vi "(Sub) Falling Step.vi"(7 "State":T1(ring), 8 "error in (no error)":errorcluster caption="에러 입력(에러 없음)", 9 "G3. Rising Step":dbl[](array[numeric]), 10 "G2. Rising Step":dbl[](array[numeric]), 11 "G1. Rising Step":dbl[](array[numeric])) -> (0 "error out":errorcluster caption="에러 출력", 1 "G3. Falling Step":dbl[](array[numeric]), 2 "G2. Falling Step":dbl[](array[numeric]), 3 "G1. Falling Step":dbl[](array[numeric]))   [LabVIEW 2017]
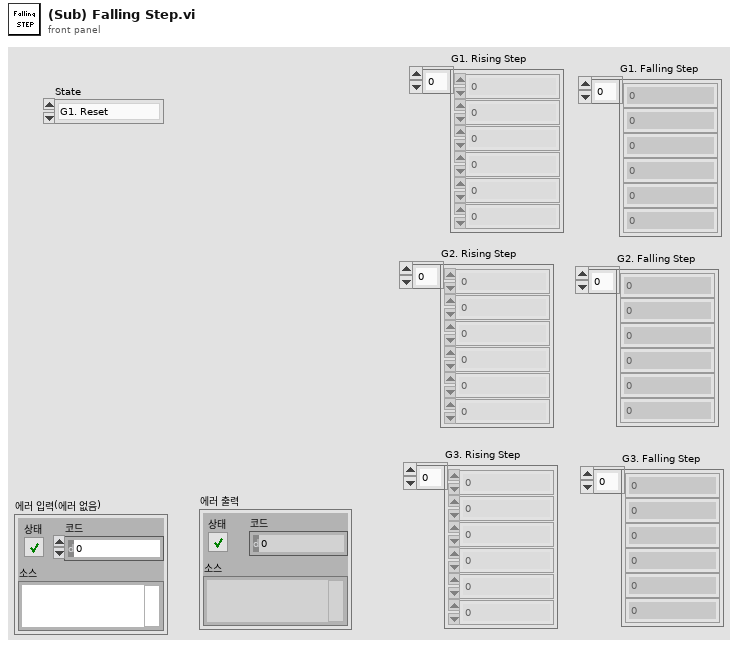
[diagram p1: front panel]
types:
  T1 = enum16{"G1. Reset", "G2. Reset", "G3. Reset", "G1. Save", "G2. Save", "G3. Save", "G1. Load", "G2. Load", "G3. Load"}
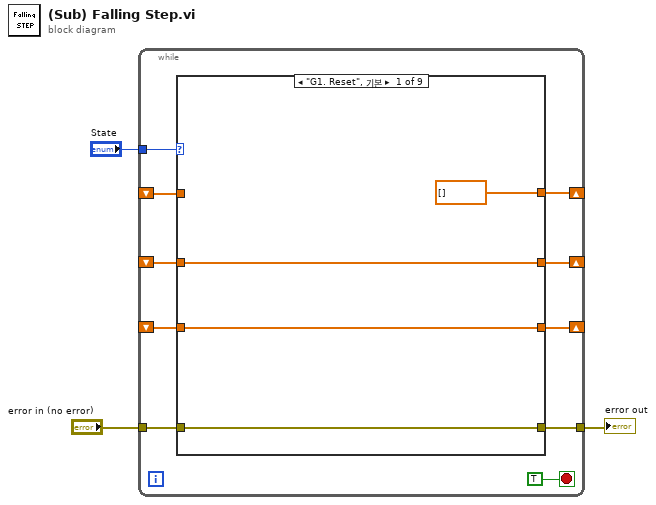
[diagram p0: block diagram]
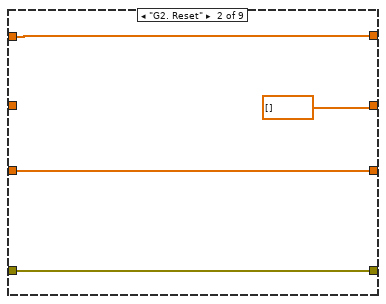
[diagram p2: hidden frame]
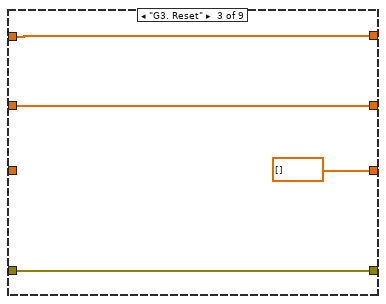
[diagram p3: hidden frame]
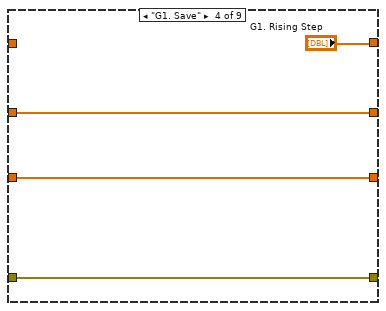
[diagram p4: hidden frame]
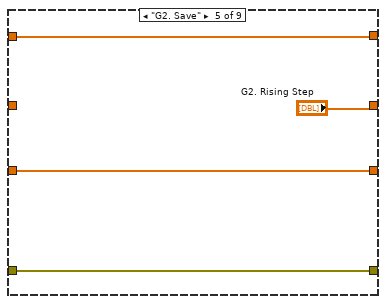
[diagram p5: hidden frame]
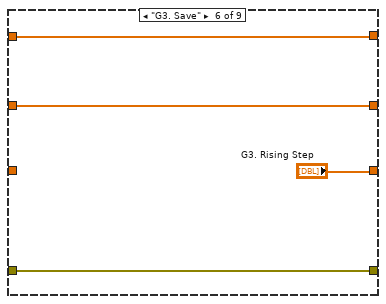
[diagram p6: hidden frame]
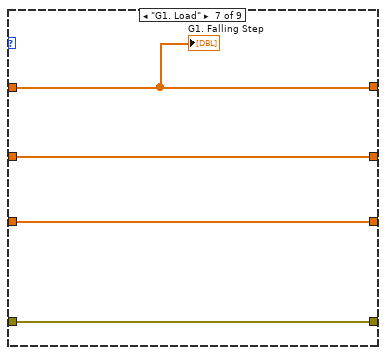
[diagram p7: hidden frame]
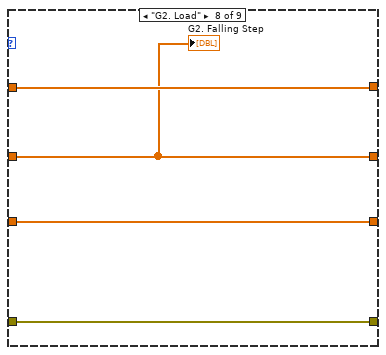
[diagram p8: hidden frame]
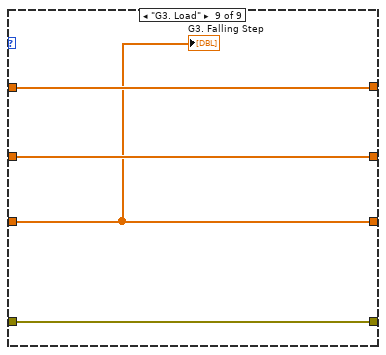
[diagram p9: hidden frame]
diagram:
  n1 = while {
    tunnel: "State" -> [w12]
    shift-right: [w11] -> _
    shift-left: _ -> [w6]
    shift-right: [w9] -> _
    shift-left: _ -> [w10]
    shift-right: [w7] -> _
    shift-left: _ -> [w8]
    tunnel: "error in (no error)" -> [w5]
    tunnel: [w4] -> w1
    stop <- TRUE stop-if-true
    n2 = case shown="\"G1. Reset\", 기본" w12 {
      tunnel: [dbl[] [] w19 w25 "G1. Rising Step" w30 w36 w38 w43 w48] -> w11
      tunnel: w10 -> [w16 _ w23 w28 _ w34 w40 w42 w47]
      tunnel: [w16 dbl[] [] w23 w28 "G2. Rising Step" w34 w40 w42 w47] -> w9
      tunnel: w8 -> [w15 w21 _ w27 w33 _ w39 w44 w46]
      tunnel: [w15 w21 dbl[] [] w27 w33 "G3. Rising Step" w39 w44 w46] -> w7
      tunnel: w6 -> [_ w19 w25 _ w30 w36 w38 w43 w48]
      tunnel: w5 -> [w14 w18 w22 w26 w32 w37 w41 w45 w49]
      tunnel: [w14 w18 w22 w26 w32 w37 w41 w45 w49] -> w4
      frame "G1. Reset", Default {
      }
      frame "G2. Reset" {
      }
      frame "G3. Reset" {
      }
      frame "G1. Save" {
      }
      frame "G2. Save" {
      }
      frame "G3. Save" {
      }
      frame "G1. Load" {
        "G1. Falling Step" <- w38
      }
      frame "G2. Load" {
        "G2. Falling Step" <- w42
      }
      frame "G3. Load" {
        "G3. Falling Step" <- w46
      }
    }
  }
  "error out" <- w1
